vi "LP Filter Metrics.vi"() -> ()   [LabVIEW 2019]
panel:
  out "XY Graph 9":cluster{dbl[], dbl[]}[](graph)=[{[1591.5494309189535, 159.15494309189532, 15.915494309189533, 1.5915494309189535, 0.15915494309189535, 0.015915494309189534, 0.0015915494309189533], [495.20998273974345, 62.4229271880735, 6.248240956900394, 0.6239944736705205, 0.06151755931078814, 0.005411201053636981, 0.005411201053636981]}, {[1591.5494309189535, 159.15494309189532, 15.915494309189533, 1.5915494309189535, 0.15915494309189535, 0.015915494309189534, 0.0015915494309189533], [371.3956776627174, 46.81692220466569, 4.685930770818215, 0.46774661763014, 0.04589562814034717, 0.0038711399018682845, 0.0038711399018682845]}, {[1591.5494309189535, 159.15494309189532, 15.915494309189533, 1.5915494309189535, 0.15915494309189535, 0.015915494309189534, 0.0015915494309189533], [309.49430057164426, 39.01393130880754, 3.9047756840751426, 0.38962263434350103, 0.03808423602056431, 0.003096524200890878, 0.003096524200890878]}, {[1591.5494309189535, 159.15494309189532, 15.915494309189533, 1.5915494309189535, 0.15915494309189535, 0.015915494309189534, 0.0015915494309189533], [270.8066641476653, 34.137063450841815, 3.4165537778564654, 0.3407953602555583, 0.03320410909560028, 0.0026273275317945832, 0.0026273275317945832]}, {[1591.5494309189535, 159.15494309189532, 15.915494309189533, 1.5915494309189535, 0.15915494309189535, 0.015915494309189534, 0.0015915494309189533], [243.72553582713797, 30.723256384408266, 3.0747984352453623, 0.3066161794363722, 0.029787236245632936, 0.002292347323821602, 0.002292347323821602]}, {[1591.5494309189535, 159.15494309189532, 15.915494309189533, 1.5915494309189535, 0.15915494309189535, 0.015915494309189534, 0.0015915494309189533], [223.41478006854084, 28.162901267388566, 2.818481944562892, 0.280981955447431, 0.027226067256090846, 0.002051657977834849, 0.002051657977834849]}, {[1591.5494309189535, 159.15494309189532, 15.915494309189533, 1.5915494309189535, 0.15915494309189535, 0.015915494309189534, 0.0015915494309189533], [207.4563743543134, 26.151193765188, 2.617090407395517, 0.2608406885772801, 0.02521290661445163, 0.0018563064603065826, 0.0018563064603065826]}, {[1591.5494309189535, 159.15494309189532, 15.915494309189533, 1.5915494309189535, 0.15915494309189535, 0.015915494309189534, 0.0015915494309189533], [194.49019515799765, 24.516681471943965, 2.4534597968174388, 0.24447604364472594, 0.023578442690996026, 0.0017059341570062516, 0.0017059341570062516]}, {[1591.5494309189535, 159.15494309189532, 15.915494309189533, 1.5915494309189535, 0.15915494309189535, 0.015915494309189534, 0.0015915494309189533], [183.68506137802152, 23.15458792453259, 2.3171009461712795, 0.23083875181365865, 0.02221560141426528, 0.00157492466432026, 0.00157492466432026]}]
  out "XY Graph 8":cluster{dbl[], dbl[]}[](graph)
  out "XY Graph 7":cluster{dbl[], dbl[]}[](graph)=[{[1591.5494309189535, 159.15494309189532, 15.915494309189533, 1.5915494309189535, 0.15915494309189535, 0.015915494309189534, 0.0015915494309189533], [1591.5494309189535, 159.15494309189532, 15.915494309189533, 1.5915494309189535, 0.15915494309189535, 0.015915494309189534, 0.0015915494309189533]}, {[1591.5494309189535, 159.15494309189532, 15.915494309189533, 1.5915494309189535, 0.15915494309189535, 0.015915494309189534, 0.0015915494309189533], [1591.5494309189535, 159.15494309189532, 15.915494309189533, 1.5915494309189535, 0.15915494309189535, 0.015915494309189534, 0.0015915494309189533]}, {[1591.5494309189535, 159.15494309189532, 15.915494309189533, 1.5915494309189535, 0.15915494309189535, 0.015915494309189534, 0.0015915494309189533], [1591.5494309189535, 159.15494309189532, 15.915494309189533, 1.5915494309189535, 0.15915494309189535, 0.015915494309189534, 0.0015915494309189533]}, {[1591.5494309189535, 159.15494309189532, 15.915494309189533, 1.5915494309189535, 0.15915494309189535, 0.015915494309189534, 0.0015915494309189533], [1591.5494309189535, 159.15494309189532, 15.915494309189533, 1.5915494309189535, 0.15915494309189535, 0.015915494309189534, 0.0015915494309189533]}, {[1591.5494309189535, 159.15494309189532, 15.915494309189533, 1.5915494309189535, 0.15915494309189535, 0.015915494309189534, 0.0015915494309189533], [1591.5494309189535, 159.15494309189532, 15.915494309189533, 1.5915494309189535, 0.15915494309189535, 0.015915494309189534, 0.0015915494309189533]}, {[1591.5494309189535, 159.15494309189532, 15.915494309189533, 1.5915494309189535, 0.15915494309189535, 0.015915494309189534, 0.0015915494309189533], [1591.5494309189535, 159.15494309189532, 15.915494309189533, 1.5915494309189535, 0.15915494309189535, 0.015915494309189534, 0.0015915494309189533]}, {[1591.5494309189535, 159.15494309189532, 15.915494309189533, 1.5915494309189535, 0.15915494309189535, 0.015915494309189534, 0.0015915494309189533], [1591.5494309189535, 159.15494309189532, 15.915494309189533, 1.5915494309189535, 0.15915494309189535, 0.015915494309189534, 0.0015915494309189533]}, {[1591.5494309189535, 159.15494309189532, 15.915494309189533, 1.5915494309189535, 0.15915494309189535, 0.015915494309189534, 0.0015915494309189533], [1591.5494309189535, 159.15494309189532, 15.915494309189533, 1.5915494309189535, 0.15915494309189535, 0.015915494309189534, 0.0015915494309189533]}, {[1591.5494309189535, 159.15494309189532, 15.915494309189533, 1.5915494309189535, 0.15915494309189535, 0.015915494309189534, 0.0015915494309189533], [1591.5494309189535, 159.15494309189532, 15.915494309189533, 1.5915494309189535, 0.15915494309189535, 0.015915494309189534, 0.0015915494309189533]}]
  out "XY Graph 6":cluster{dbl[], dbl[]}[](graph)=[{[1591.5494309189535, 159.15494309189532, 15.915494309189533, 1.5915494309189535, 0.15915494309189535, 0.015915494309189534, 0.0015915494309189533], [1767.099740912122, 176.77509646524533, 17.676678810580086, 1.7667678894862797, 0.17577664872265833, 0.016638452343507144, 0.0008956632431088917]}, {[1591.5494309189535, 159.15494309189532, 15.915494309189533, 1.5915494309189535, 0.15915494309189535, 0.015915494309189534, 0.0015915494309189533], [1666.5013949938002, 166.66559537189198, 16.66567589334608, 1.6656672905453724, 0.16566590855865096, 0.015640711483454667, 0.0007115391462718495]}, {[1591.5494309189535, 159.15494309189532, 15.915494309189533, 1.5915494309189535, 0.15915494309189535, 0.015915494309189534, 0.0015915494309189533], [1633.1249729596805, 163.31938425094248, 16.331046152781898, 1.6322040848298347, 0.16231834334347942, 0.015273471245026421, 0.0006415507485982914]}, {[1591.5494309189535, 159.15494309189532, 15.915494309189533, 1.5915494309189535, 0.15915494309189535, 0.015915494309189534, 0.0015915494309189533], [1617.9870361484807, 161.80244348926595, 16.17934893355119, 1.6170344814424644, 0.1608011553281375, 0.015126362044504297, 0.0005597638020751991]}, {[1591.5494309189535, 159.15494309189532, 15.915494309189533, 1.5915494309189535, 0.15915494309189535, 0.015915494309189534, 0.0015915494309189533], [1609.8449378687549, 160.98669739729402, 16.09777278146849, 1.608876591490976, 0.15998427250574704, 0.01501341797724548, 0.0005410281358335853]}, {[1591.5494309189535, 159.15494309189532, 15.915494309189533, 1.5915494309189535, 0.15915494309189535, 0.015915494309189534, 0.0015915494309189533], [1604.9628114166244, 160.49761135922873, 16.04886327886417, 1.6039855779052405, 0.1594937978511623, 0.014979592854989706, 0.000488757868653753]}, {[1591.5494309189535, 159.15494309189532, 15.915494309189533, 1.5915494309189535, 0.15915494309189535, 0.015915494309189534, 0.0015915494309189533], [1601.8050566605493, 160.18128906323892, 16.017230494249855, 1.6008223170852807, 0.1591757267331502, 0.014916206222619148, 0.0004311266700662223]}, {[1591.5494309189535, 159.15494309189532, 15.915494309189533, 1.5915494309189535, 0.15915494309189535, 0.015915494309189534, 0.0015915494309189533], [1599.6450662690663, 159.96492391147012, 15.9955936144505, 1.598658482860332, 0.15895977041310844, 0.014913270116707266, 0.00044571712858833496]}, {[1591.5494309189535, 159.15494309189532, 15.915494309189533, 1.5915494309189535, 0.15915494309189535, 0.015915494309189534, 0.0015915494309189533], [1598.102505316461, 159.81041021148107, 15.980141944847217, 1.5971131797141296, 0.15880336850266868, 0.014867311942267088, 0.00045600528696067044]}]
  out "XY Graph 5":cluster{dbl[], dbl[]}[](graph)
  out "XY Graph 4":cluster{dbl[], dbl[]}[](graph)=[{[1591.5494309189535, 159.15494309189532, 15.915494309189533, 1.5915494309189535, 0.15915494309189535, 0.015915494309189534, 0.0015915494309189533], [1591.5494309189535, 159.15494309189532, 15.915494309189533, 1.5915494309189535, 0.15915494309189535, 0.015915494309189534, 0.0015915494309189533]}, {[1591.5494309189535, 159.15494309189532, 15.915494309189533, 1.5915494309189535, 0.15915494309189535, 0.015915494309189534, 0.0015915494309189533], [1591.5494309189535, 159.15494309189532, 15.915494309189533, 1.5915494309189535, 0.15915494309189535, 0.015915494309189534, 0.0015915494309189533]}, {[1591.5494309189535, 159.15494309189532, 15.915494309189533, 1.5915494309189535, 0.15915494309189535, 0.015915494309189534, 0.0015915494309189533], [1591.5494309189535, 159.15494309189532, 15.915494309189533, 1.5915494309189535, 0.15915494309189535, 0.015915494309189534, 0.0015915494309189533]}, {[1591.5494309189535, 159.15494309189532, 15.915494309189533, 1.5915494309189535, 0.15915494309189535, 0.015915494309189534, 0.0015915494309189533], [1591.5494309189535, 159.15494309189532, 15.915494309189533, 1.5915494309189535, 0.15915494309189535, 0.015915494309189534, 0.0015915494309189533]}, {[1591.5494309189535, 159.15494309189532, 15.915494309189533, 1.5915494309189535, 0.15915494309189535, 0.015915494309189534, 0.0015915494309189533], [1591.5494309189535, 159.15494309189532, 15.915494309189533, 1.5915494309189535, 0.15915494309189535, 0.015915494309189534, 0.0015915494309189533]}, {[1591.5494309189535, 159.15494309189532, 15.915494309189533, 1.5915494309189535, 0.15915494309189535, 0.015915494309189534, 0.0015915494309189533], [1591.5494309189535, 159.15494309189532, 15.915494309189533, 1.5915494309189535, 0.15915494309189535, 0.015915494309189534, 0.0015915494309189533]}, {[1591.5494309189535, 159.15494309189532, 15.915494309189533, 1.5915494309189535, 0.15915494309189535, 0.015915494309189534, 0.0015915494309189533], [1591.5494309189535, 159.15494309189532, 15.915494309189533, 1.5915494309189535, 0.15915494309189535, 0.015915494309189534, 0.0015915494309189533]}, {[1591.5494309189535, 159.15494309189532, 15.915494309189533, 1.5915494309189535, 0.15915494309189535, 0.015915494309189534, 0.0015915494309189533], [1591.5494309189535, 159.15494309189532, 15.915494309189533, 1.5915494309189535, 0.15915494309189535, 0.015915494309189534, 0.0015915494309189533]}, {[1591.5494309189535, 159.15494309189532, 15.915494309189533, 1.5915494309189535, 0.15915494309189535, 0.015915494309189534, 0.0015915494309189533], [1591.5494309189535, 159.15494309189532, 15.915494309189533, 1.5915494309189535, 0.15915494309189535, 0.015915494309189534, 0.0015915494309189533]}]
  out "1/RC":T1(graph)
  out "Butterworth Filters":T1(graph)
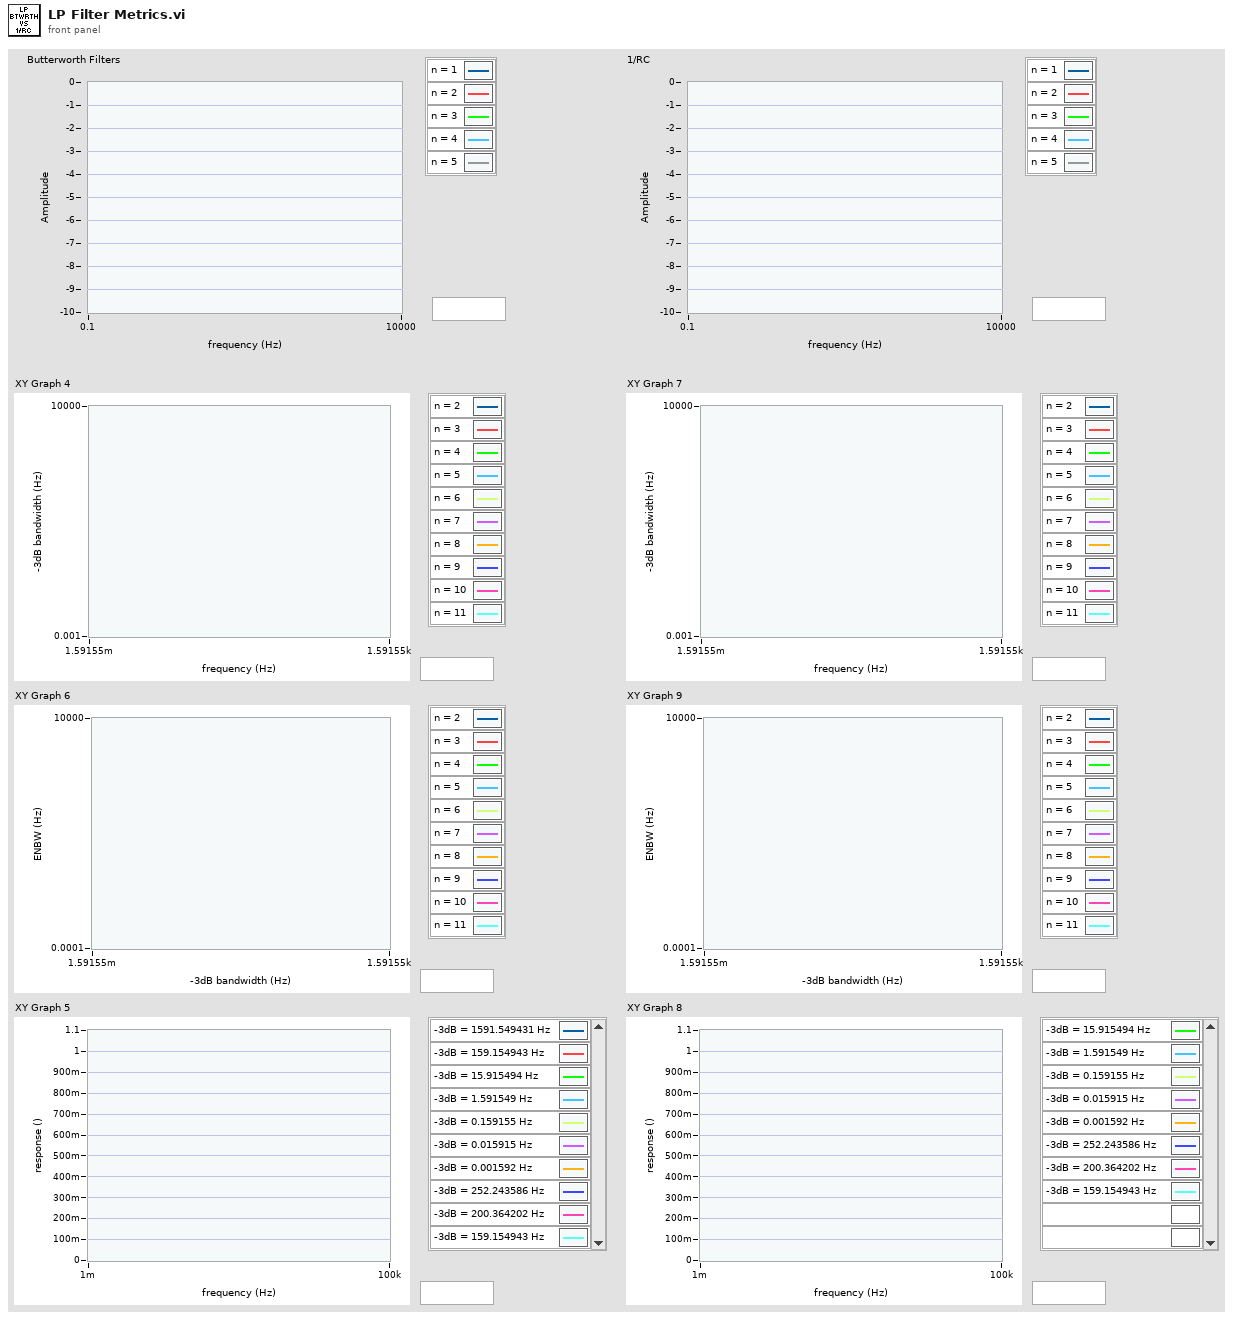
[diagram p1: front panel]
types:
  T1 = cluster{"Ramp Pattern":dbl[], "magnitude":dbl[]}[]
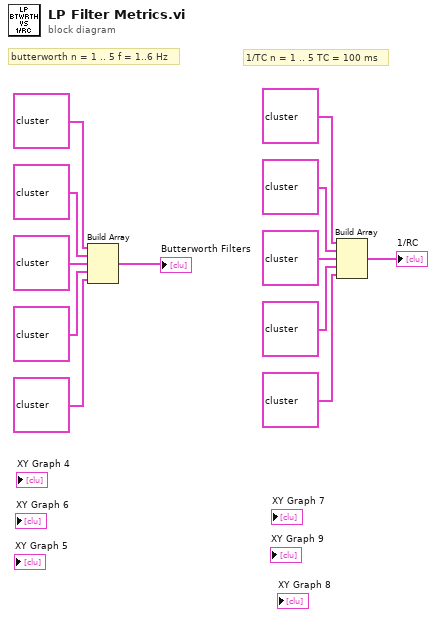
[diagram p0: block diagram]
diagram:
  # "1/TC n = 1 .. 5 TC = 100 ms"
  # "butterworth n = 1 .. 5 f = 1..6 Hz"
  n1 = Build Array(cluster{"Ramp Pattern":dbl[], "magnitude":dbl[]} {"Ramp Pattern"=array[1000 elements], "magnitude"=array[1000 elements]} ("XY Graph"), cluster{"Ramp Pattern":dbl[], "magnitude":dbl[]} {"Ramp Pattern"=array[1000 elements], "magnitude"=array[1000 elements]} ("XY Graph"), cluster{"Ramp Pattern":dbl[], "magnitude":dbl[]} {"Ramp Pattern"=array[1000 elements], "magnitude"=array[1000 elements]} ("XY Graph"), cluster{"Ramp Pattern":dbl[], "magnitude":dbl[]} {"Ramp Pattern"=array[1000 elements], "magnitude"=array[1000 elements]} ("XY Graph"), cluster{"Ramp Pattern":dbl[], "magnitude":dbl[]} {"Ramp Pattern"=array[1000 elements], "magnitude"=array[1000 elements]} ("XY Graph")) -> (→"Butterworth Filters":T1)
  n2 = Build Array(cluster{"Ramp Pattern":dbl[], "magnitude":dbl[]} {"Ramp Pattern"=array[1000 elements], "magnitude"=array[1000 elements]} ("XY Graph"), cluster{"Ramp Pattern":dbl[], "magnitude":dbl[]} {"Ramp Pattern"=array[1000 elements], "magnitude"=array[1000 elements]} ("XY Graph"), cluster{"Ramp Pattern":dbl[], "magnitude":dbl[]} {"Ramp Pattern"=array[1000 elements], "magnitude"=array[1000 elements]} ("XY Graph"), cluster{"Ramp Pattern":dbl[], "magnitude":dbl[]} {"Ramp Pattern"=array[1000 elements], "magnitude"=array[1000 elements]} ("XY Graph"), cluster{"Ramp Pattern":dbl[], "magnitude":dbl[]} {"Ramp Pattern"=array[1000 elements], "magnitude"=array[1000 elements]} ("XY Graph")) -> (→"1/RC":T1)
